vi "RSZVB Set Source Power Calibration State.vi"(8 "error in (no error)":errorcluster {"code" format="%.0x"}, 10 "Calibration State (T: On)":bool=TRUE, 11 "VISA session":refnum<visa-resource-name>) -> (0 "error out":errorcluster {"code" format="%.0x"}, 3 "dup VISA session":refnum<visa-resource-name>)   [LabVIEW 2011]
doc: "This VI enables or disables the source power calibration. \n\nNotes:\n\n(1) It is not possible to disable flatness calibration and the reference receiver calibration simultaneously.\n\nRemote-control command(s):\nSOURce<Ch>:POWer:CORRection:COLLect:FLATness ON | OFF"
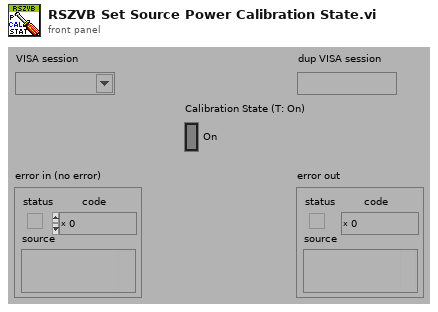
[diagram p1: front panel]
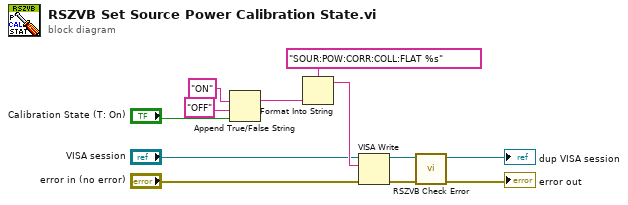
[diagram p0: block diagram]
diagram:
  n1 = Append True/False String(1:"Calibration State (T: On)", 2:"OFF", 3:"ON") -> (0:w6:string)  [unwired: 1 in]
  n2 = Format Into String(format string="SOUR:POW:CORR:COLL:FLAT %s", w6) -> (resulting string=w9:string)  [unwired: 2 in, 1 out]
  n3 = VISA Write(VISA resource name="VISA session", write buffer=w9, error in (no error)="error in (no error)") -> (VISA resource name out=w10:refnum<visa-resource-name>, error out=w11:errorcluster)  [unwired: 1 out]
  n4 = call "RSZVB Check Error.vi"("error in (no error)"=w11, "VISA session"=w10) -> ("error out"=→"error out":errorcluster, "dup VISA session"=→"dup VISA session":refnum<visa-resource-name>)  [unwired: 8 in]
